vi "Cambio de unidades.vi"() -> ()   [LabVIEW 2010]
panel:
  out "Thermometer":dbl(slide) scale=0.0..100.0
  in  "stop":bool
  out "Numeric 2":dbl
  in  "Numeric":dbl
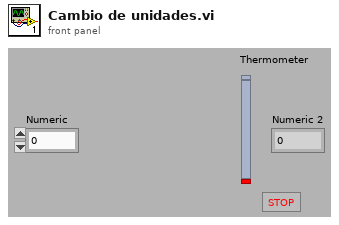
[diagram p1: front panel]
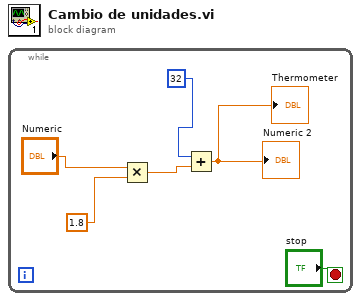
[diagram p0: block diagram]
diagram:
  n1 = while {
    stop <- "stop" stop-if-true
    n2 = Multiply(x="Numeric", y=1.8) -> (x*y=w4:dbl)
    n3 = Add(x=32, y=w4) -> (x+y=→"Numeric 2" →"Thermometer":dbl)
  }
